vi "_Build_Cluster_Query.vi"(8 "error in (no error)":errorcluster, 11 "Postgres Connector In":refnum<class "Postgres Connector.lvclass">) -> (0 "error out":errorcluster, 1 "State After Query":string, 2 "Query Return":T1)   [LabVIEW 2019, in "PG_LIB.lvlib" / "Postgres Connector.lvclass"]
doc: "This VI build the cluster containing the important information of the query"
uses:
  Postgres Connector.lvclass
  Cluster_Return_Of_The_Query.ctl
  Postgres Connector.lvclass/Postgres Connector.ctl
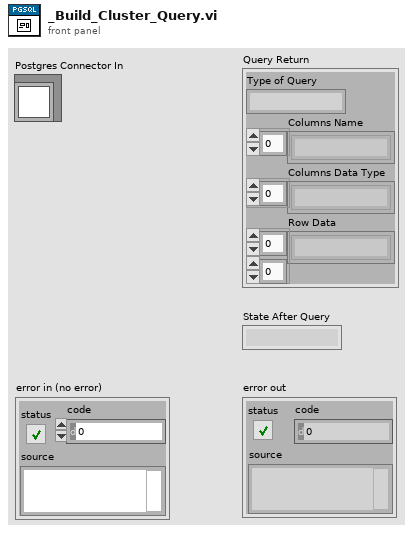
[diagram p1: front panel]
types:
  T1 = typedef "PG_LIB.lvlib/Postgres Connector.lvclass/Cluster_Return_Of_The_Query.ctl" = cluster{"Type of Query":string, "Columns Name":string[], "Columns Data Type":string[], "Row Data":string[][]}
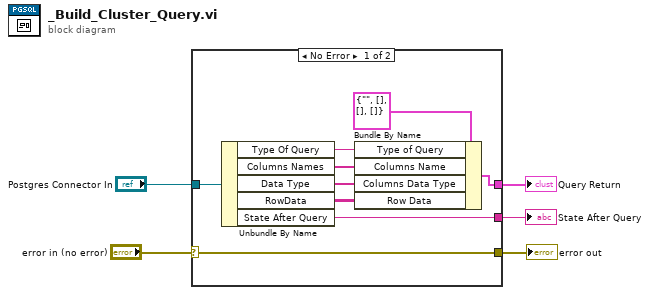
[diagram p0: block diagram]
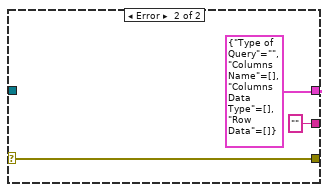
[diagram p2: hidden frame]
diagram:
  n1 = case shown="No Error" "error in (no error)" {
    selector: "error in (no error)" -> [w12 w17]
    tunnel: [w13 T1 {"Type of Query"="", "Columns Name"=[], "Columns Data Type"=[], "Row Data"=[]}] -> w5
    tunnel: [w12 w17] -> w3
    tunnel: "Postgres Connector In" -> [w11 _]
    tunnel: [w7 "" ("State After Query")] -> w1
    frame No Error {
      n2 = Unbundle By Name(w11) -> ("Type Of Query"=w6:string, "Columns Names"=w8:string[], "Data Type"=w10:string[], "RowData"=w9:string[][], "State After Query"=w7:string)
      n3 = Bundle By Name(cluster=T1 {"Type of Query"="", "Columns Name"=[], "Columns Data Type"=[], "Row Data"=[]}, "Type of Query"=w6, "Columns Name"=w8, "Columns Data Type"=w10, "Row Data"=w9) -> (w13:T1)
    }
    frame Error {
    }
  }
  "error out" <- w3
  "Query Return" <- w5
  "State After Query" <- w1
